vi "Init.vi"(10 "Spawn":T1) -> (3 "Base Spawn out":refnum<class "Base Spawn.lvclass">)   [LabVIEW 2025, in "jettl.lvlib" / "Spawn.lvlib" / "Base Spawn.lvclass"]
uses:
  Base Spawn.lvclass
  Spawn.ctl
  Attributes/Attributes/Attributes.lvclass
  Transport/Transport/Transport.lvclass
  Base Spawn.lvclass/Base Spawn.ctl
  Spawn.lvlib
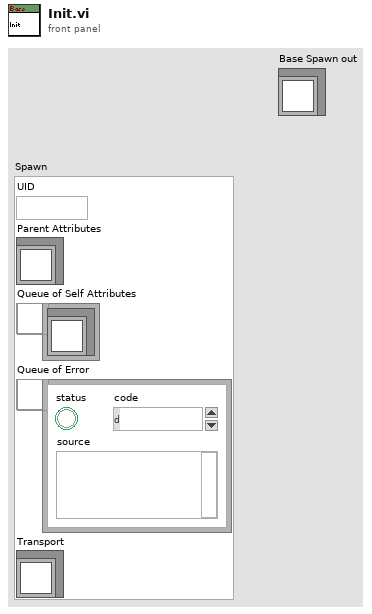
[diagram p1: front panel]
types:
  T1 = typedef "jettl.lvlib/Spawn.lvlib/Spawn.ctl" = cluster{"UID":string, "Parent Attributes":refnum<class "Attributes.lvclass">, "Queue of Self Attributes":refnum<queue>, "Queue of Error":refnum<queue>, "Transport":refnum<class "Transport.lvclass">}
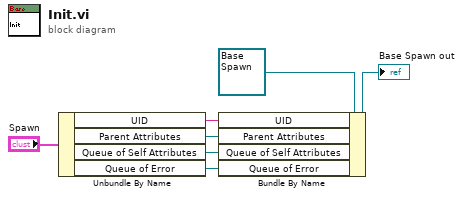
[diagram p0: block diagram]
diagram:
  n1 = Unbundle By Name("Spawn") -> ("UID"=w4:string, "Parent Attributes"=w3:refnum<class "Attributes.lvclass">, "Queue of Self Attributes"=w2:refnum<queue>, "Queue of Error"=w1:refnum<queue>)
  n2 = Bundle By Name(cluster=refnum<class "Base Spawn.lvclass"> refnum ("Base Spawn out"), "UID"=w4, "Parent Attributes"=w3, "Queue of Self Attributes"=w2, "Queue of Error"=w1) -> (→"Base Spawn out":refnum<class "Base Spawn.lvclass">)
